vi "getposition.vi"(0 "string":string) -> (1 "READ":string, 2 "x-position":dbl, 3 "y-position":dbl, 4 "z-position":dbl)   [LabVIEW 2016]
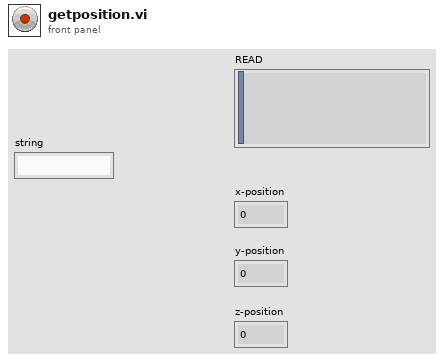
[diagram p1: front panel]
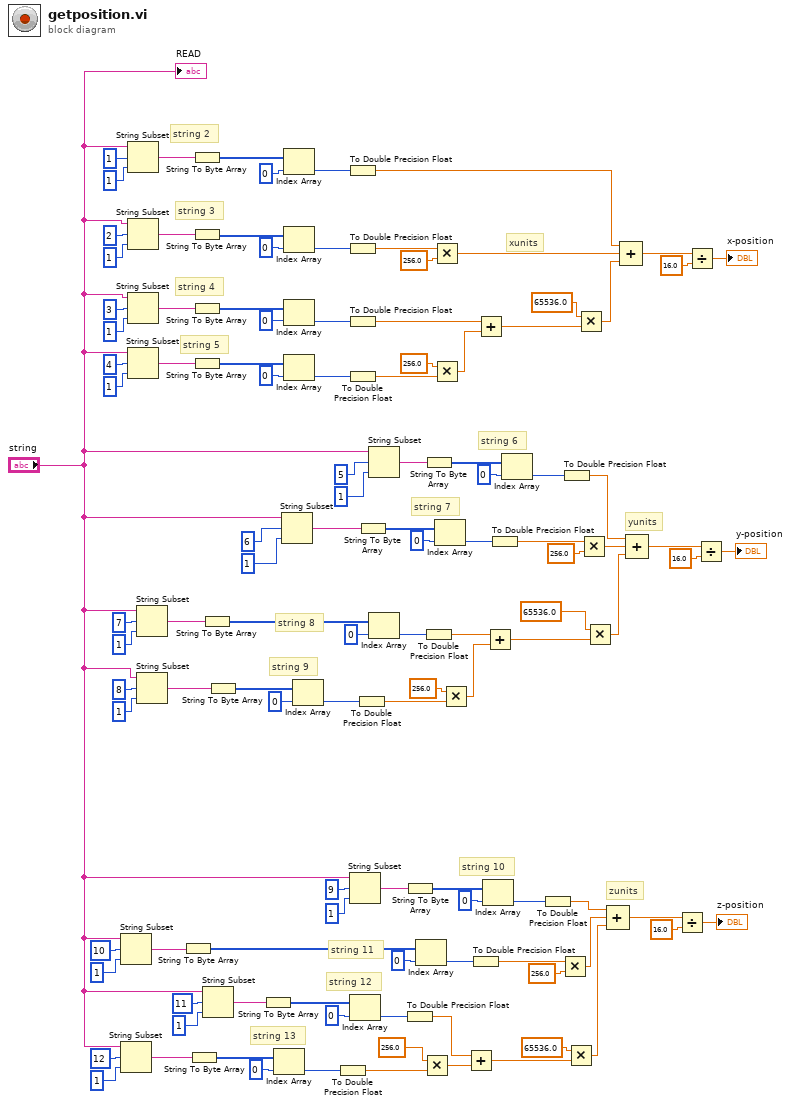
[diagram p0: block diagram]
diagram:
  # "zunits"
  # "string 13"
  # "string 12"
  # "string 11"
  # "string 10"
  # "yunits"
  # "string 9"
  # "string 8"
  # "string 7"
  # "string 6"
  # "xunits"
  # "string 5"
  # "string 4"
  # "string 3"
  # "string 2"
  n1 = String Subset(string="string", offset (0)=10, length (rest)=1 ("length (rest)")) -> (substring=w32:string)
  n2 = String Subset(string="string", offset (0)=12, length (rest)=1 ("length (rest)")) -> (substring=w22:string)
  n3 = String Subset(string="string", offset (0)=1, length (rest)=1 ("length (rest)")) -> (substring=w113:string)
  n4 = String Subset(string="string", offset (0)=2, length (rest)=1 ("length (rest)")) -> (substring=w108:string)
  n5 = String Subset(string="string", offset (0)=3, length (rest)=1 ("length (rest)")) -> (substring=w103:string)
  n6 = String Subset(string="string", offset (0)=4, length (rest)=1 ("length (rest)")) -> (substring=w98:string)
  n7 = String Subset(string="string", offset (0)=7, length (rest)=1 ("length (rest)")) -> (substring=w65:string)
  n8 = String Subset(string="string", offset (0)=8, length (rest)=1 ("length (rest)")) -> (substring=w60:string)
  n9 = String To Byte Array(string=w32) -> (unsigned byte array=w31:u8[])
  n10 = String To Byte Array(string=w22) -> (unsigned byte array=w21:u8[])
  n11 = String To Byte Array(string=w113) -> (unsigned byte array=w112:u8[])
  n12 = String To Byte Array(string=w108) -> (unsigned byte array=w107:u8[])
  n13 = String To Byte Array(string=w103) -> (unsigned byte array=w102:u8[])
  n14 = String To Byte Array(string=w98) -> (unsigned byte array=w97:u8[])
  n15 = String To Byte Array(string=w65) -> (unsigned byte array=w64:u8[])
  n16 = String Subset(string="string", offset (0)=11, length (rest)=1 ("length (rest)")) -> (substring=w27:string)
  n17 = String To Byte Array(string=w60) -> (unsigned byte array=w59:u8[])
  n18 = String To Byte Array(string=w27) -> (unsigned byte array=w26:u8[])
  n19 = Index Array(array=w21, index=0) -> (element=w17:u8)
  n20 = String Subset(string="string", offset (0)=6, length (rest)=1 ("length (rest)")) -> (substring=w70:string)
  n21 = Index Array(array=w112, index=0) -> (element=w84:u8)
  n22 = Index Array(array=w107, index=0) -> (element=w87:u8)
  n23 = Index Array(array=w102, index=0) -> (element=w89:u8)
  n24 = Index Array(array=w97, index=0) -> (element=w93:u8)
  n25 = Index Array(array=w59, index=0) -> (element=w55:u8)
  n26 = To Double Precision Float(number=w17) -> (double precision float=w16:dbl)
  n27 = To Double Precision Float(number=w84) -> (double precision float=w83:dbl)
  n28 = To Double Precision Float(number=w87) -> (double precision float=w86:dbl)
  n29 = To Double Precision Float(number=w89) -> (double precision float=w90:dbl)
  n30 = To Double Precision Float(number=w93) -> (double precision float=w92:dbl)
  n31 = String Subset(string="string", offset (0)=9, length (rest)=1 ("length (rest)")) -> (substring=w37:string)
  n32 = Index Array(array=w26, index=0) -> (element=w13:u8)
  n33 = To Double Precision Float(number=w55) -> (double precision float=w54:dbl)
  n34 = String To Byte Array(string=w70) -> (unsigned byte array=w69:u8[])
  n35 = String Subset(string="string", offset (0)=5, length (rest)=1 ("length (rest)")) -> (substring=w75:string)
  n36 = Index Array(array=w64, index=0) -> (element=w51:u8)
  n37 = String To Byte Array(string=w37) -> (unsigned byte array=w36:u8[])
  n38 = To Double Precision Float(number=w13) -> (double precision float=w14:dbl)
  n39 = Index Array(array=w31, index=0) -> (element=w11:u8)
  n40 = Multiply(x=256.0, y=w16) -> (x*y=w19:dbl)
  n41 = String To Byte Array(string=w75) -> (unsigned byte array=w74:u8[])
  n42 = To Double Precision Float(number=w51) -> (double precision float=w52:dbl)
  n43 = Multiply(x=w86, y=256.0) -> (x*y=w82:dbl)
  n44 = Multiply(x=256.0, y=w92) -> (x*y=w95:dbl)
  n45 = Index Array(array=w69, index=0) -> (element=w49:u8)
  n46 = Multiply(x=256.0, y=w54) -> (x*y=w57:dbl)
  n47 = Add(x=w14, y=w19) -> (x+y=w18:dbl)
  n48 = To Double Precision Float(number=w11) -> (double precision float=w10:dbl)
  n49 = Add(x=w90, y=w95) -> (x+y=w94:dbl)
  n50 = Index Array(array=w36, index=0) -> (element=w8:u8)
  n51 = Add(x=w52, y=w57) -> (x+y=w56:dbl)
  n52 = To Double Precision Float(number=w49) -> (double precision float=w48:dbl)
  n53 = Index Array(array=w74, index=0) -> (element=w46:u8)
  n54 = To Double Precision Float(number=w8) -> (double precision float=w7:dbl)
  n55 = Multiply(x=w10, y=256.0) -> (x*y=w6:dbl)
  n56 = To Double Precision Float(number=w46) -> (double precision float=w45:dbl)
  n57 = Multiply(x=65536.0, y=w18) -> (x*y=w5:dbl)
  n58 = Multiply(x=65536.0, y=w94) -> (x*y=w81:dbl)
  n59 = Multiply(x=w48, y=256.0) -> (x*y=w44:dbl)
  n60 = Multiply(x=65536.0, y=w56) -> (x*y=w43:dbl)
  n61 = Compound Arithmetic op=ADD(w7, w6, w5) -> (w4:dbl)
  n62 = Compound Arithmetic op=ADD(w83, w82, w81) -> (w80:dbl)
  n63 = Compound Arithmetic op=ADD(w45, w44, w43) -> (w42:dbl)
  n64 = Divide(x=w4, y=16.0 ("x")) -> (x/y=→"z-position":dbl)
  n65 = Divide(x=w80, y=16.0 ("x")) -> (x/y=→"x-position":dbl)
  n66 = Divide(x=w42, y=16.0 ("x")) -> (x/y=→"y-position":dbl)
  "READ" <- "string"
